vi "Metadata to FITS file header.vi"() -> ()   [LabVIEW 2023]
uses:
  gfitsio.lvlib
  gfitsio-write-key-double.vi
  gfitsio-write-key-string.vi
  cfitsio-bitpix.ctl
  gfitsio-read-image-subset-i16-2d.vi
  gfitsio-write-key-integer.vi
  gfitsio-write-image-subset-i16-2d.vi
  gfitsio-read-key-double.vi
  subvi/Git/GIT Data.ctl
  Data/MetaData/Typedef/MetaData.ctl
panel:
  out "concatenated string":string
  out "value":dbl
  out "header":string[](array[string])
  in  "MetaData":T1={"Test Name"="FPA CPT", "WOA Number"="0222", "User Name"="OCIfpa", "Operator"="Steve Marlow", "DUT SN"="SN0001", "Machine Name"="NI01", "OS Version"="WinNT 7", "Location"="HFF", "Top VI LV Rev."=123, "Lab Temperature"=23.5, "Lab Humidity"=49.9, "GIT"=[]}
  in  "file path":path=path "C:/Users/smarlow/Documents/FPA/gain_00014ms_1600x200_0017.fits"
  out "error out":errorcluster
  out "data":i16[][](array[numeric])
  out "Image":T3(plugin-control)
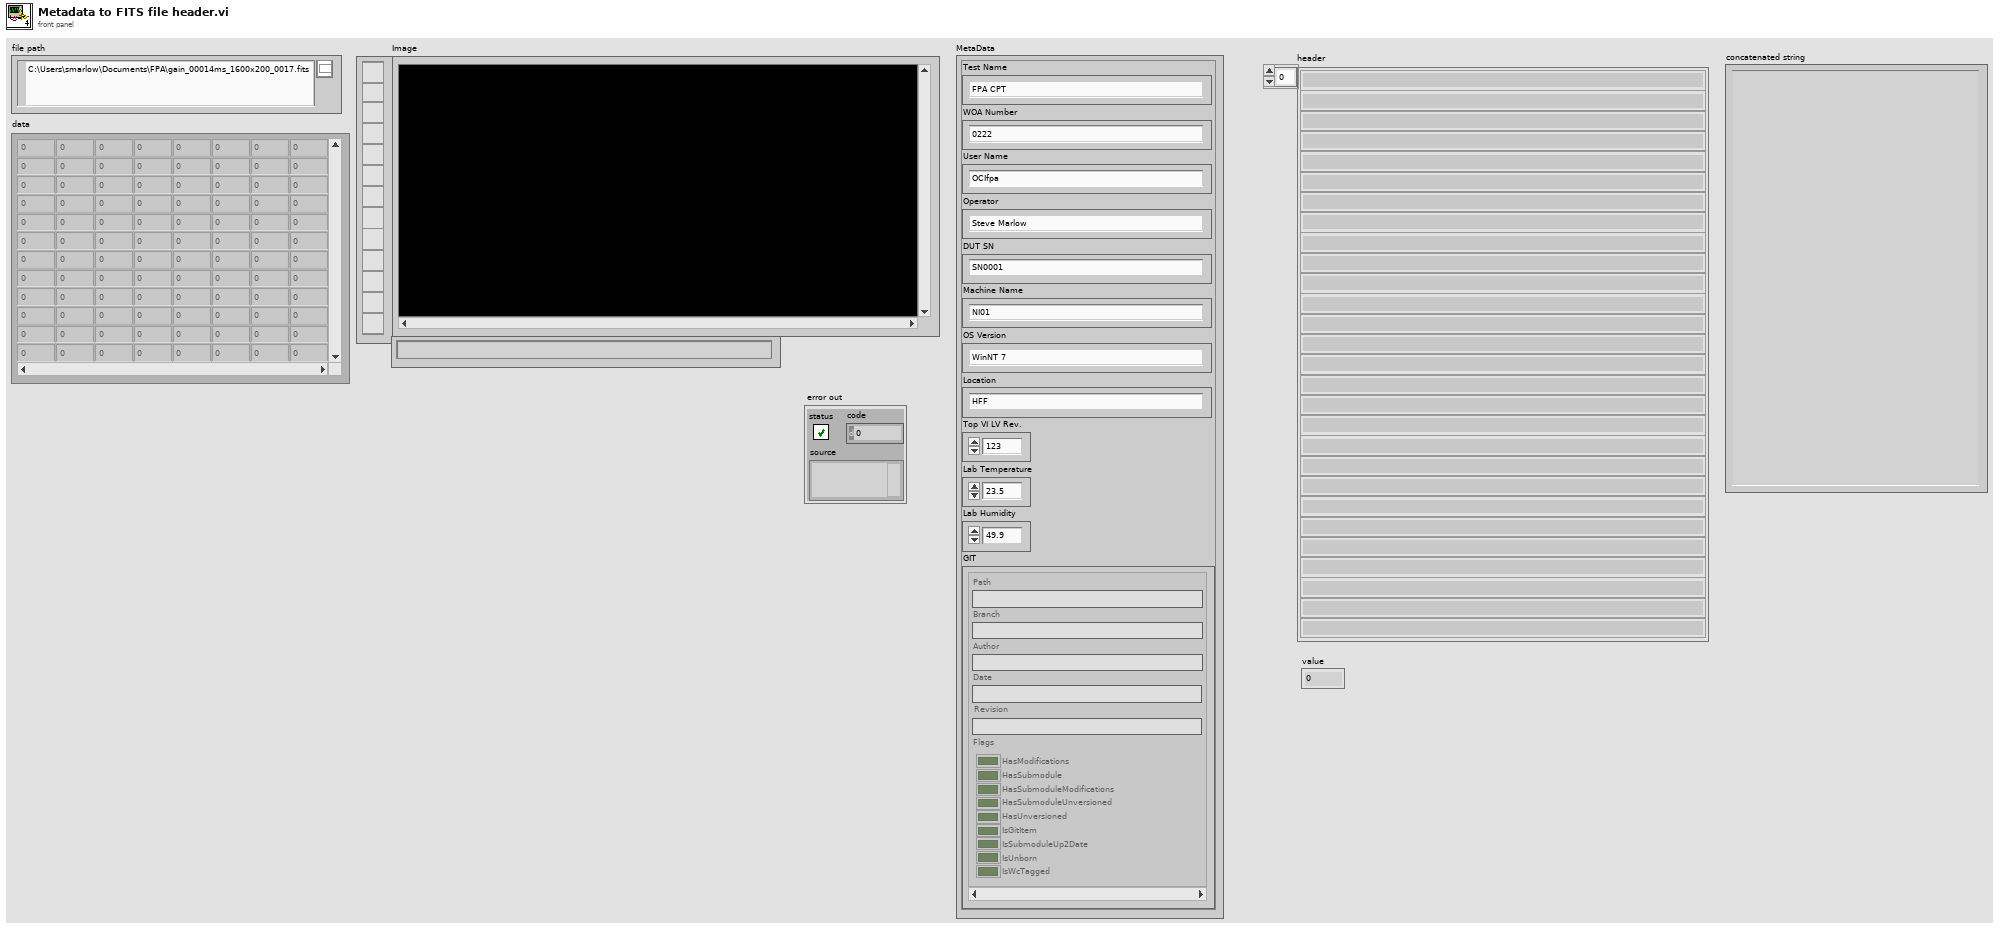
[diagram p1: front panel]
types:
  T1 = typedef "Data.MetaData.lvclass/MetaData.ctl" = cluster{"Test Name":string, "WOA Number":string, "User Name":string, "Operator":string, "DUT SN":string, "Machine Name":string, "OS Version":string, "Location":string, "Top VI LV Rev.":u32, "Lab Temperature":dbl, "Lab Humidity":dbl, "GIT":T2[]}
  T2 = typedef "GIT Data.ctl" = cluster{"Path":string, "Branch":string, "Author":string, "Date":string, "Revision":string, "Flags":cluster{"HasModifications":bool, "HasSubmodule":bool, "HasSubmoduleModifications":bool, "HasSubmoduleUnversioned":bool, "HasUnversioned":bool, "IsGitItem":bool, "IsSubmoduleUp2Date":bool, "IsUnborn":bool, "IsWcTagged":bool}}
  T3 = typedef "IMAQ Image.ctl" = refnum<image>
  T4 = typedef "gfitsio.lvlib/cfitsio-bitpix.ctl" = i32
  T5 = enum16{"open", "open or create", "create or replace", "create", "open (read only)"}
  T6 = typedef "Image Type" = u32
  T7 = typedef "gfitsio.lvlib/gfitsio-refnum.ctl" = refnum<k1>
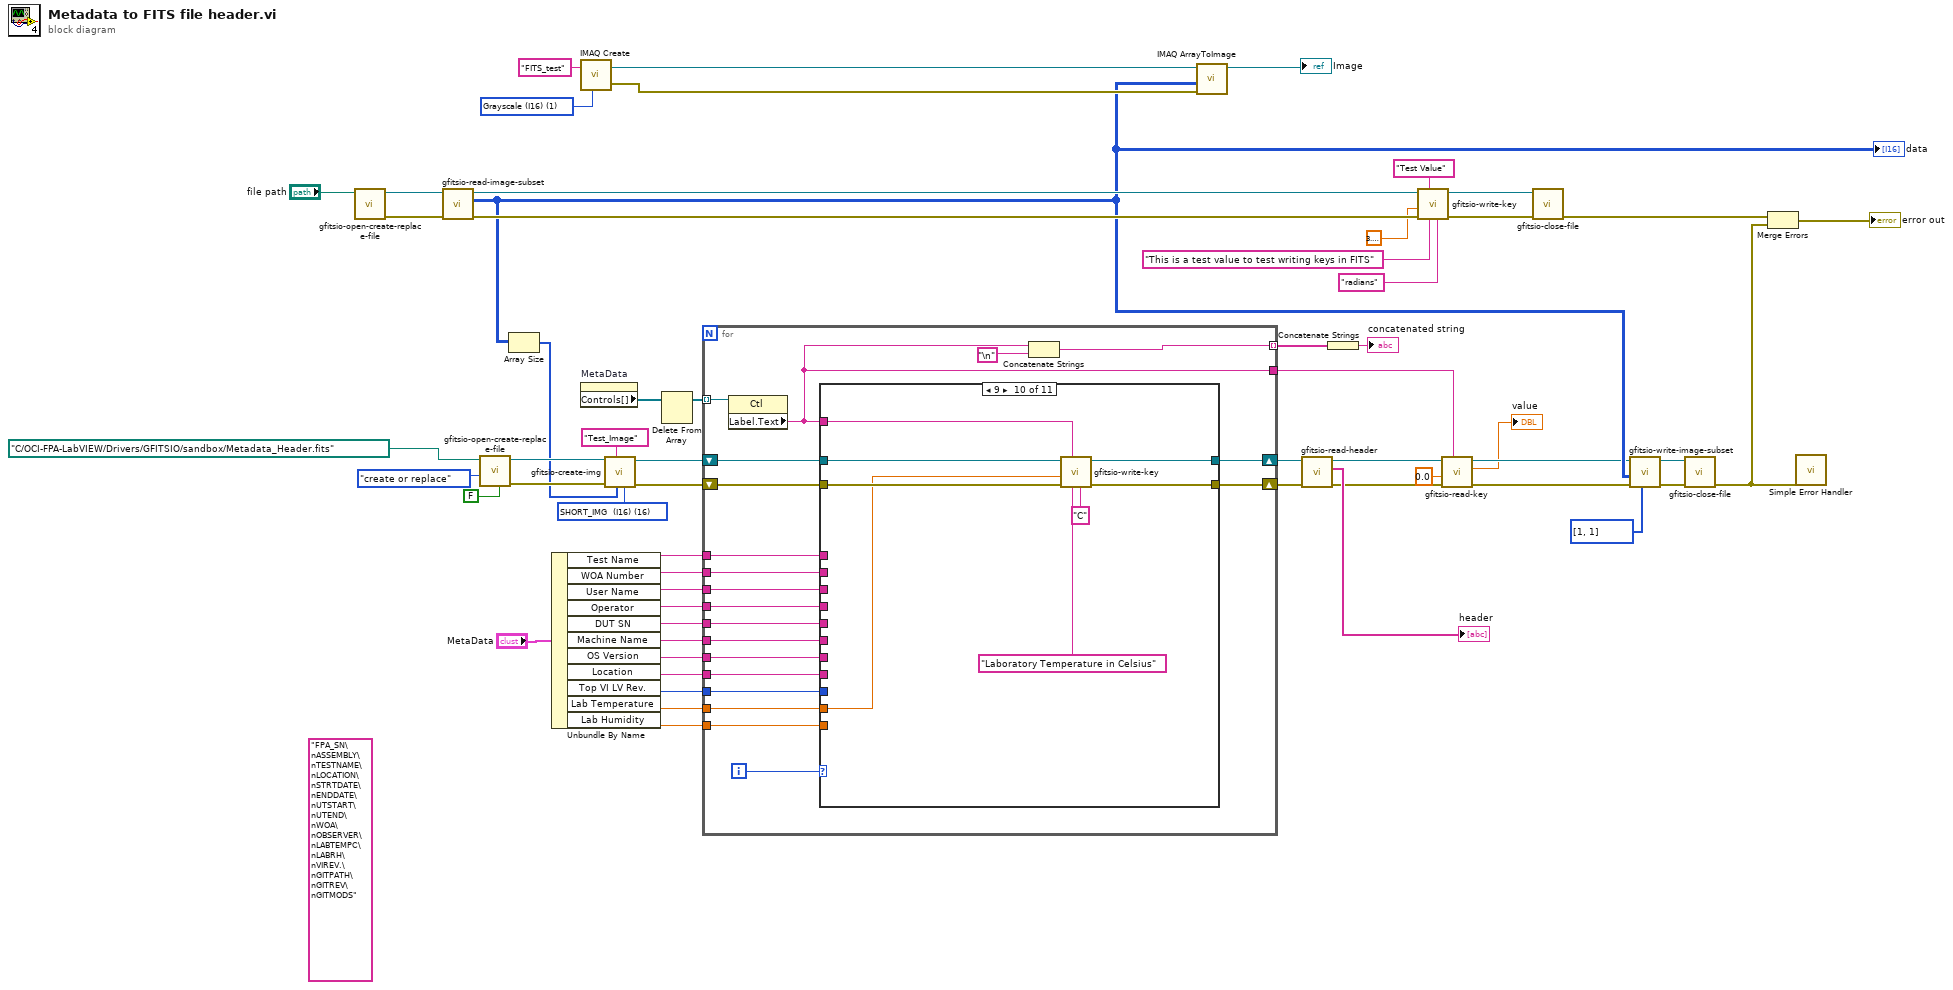
[diagram p0: block diagram]
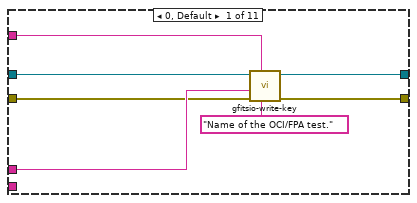
[diagram p2: hidden frame]
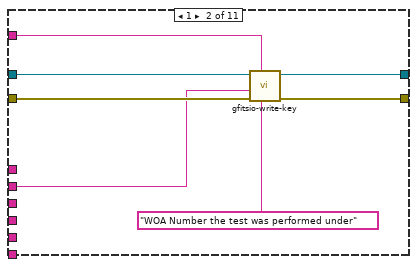
[diagram p3: hidden frame]
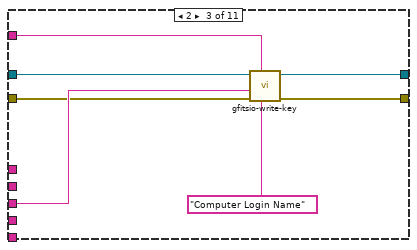
[diagram p4: hidden frame]
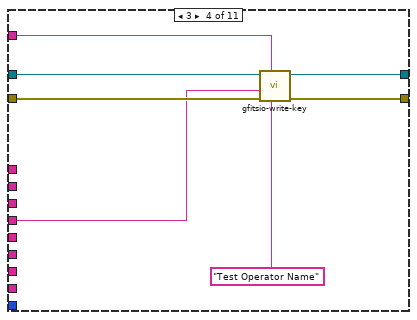
[diagram p5: hidden frame]
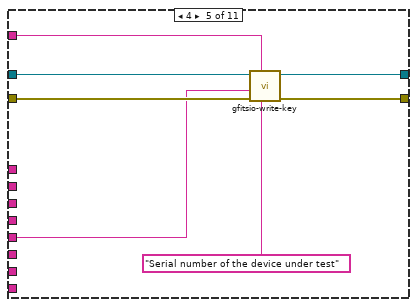
[diagram p6: hidden frame]
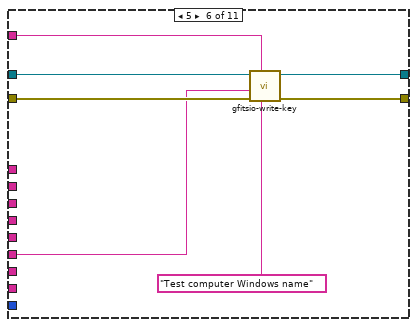
[diagram p7: hidden frame]
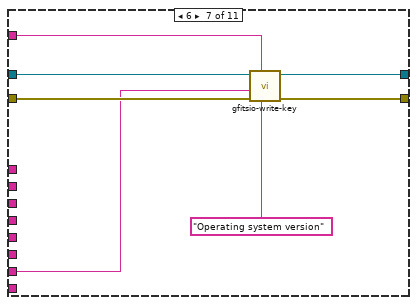
[diagram p8: hidden frame]
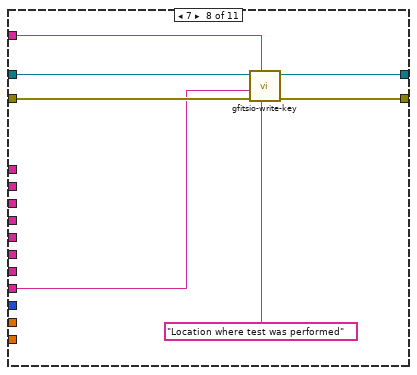
[diagram p9: hidden frame]
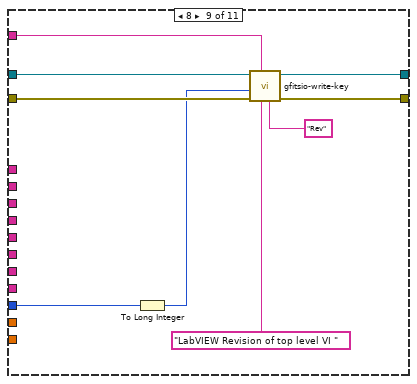
[diagram p10: hidden frame]
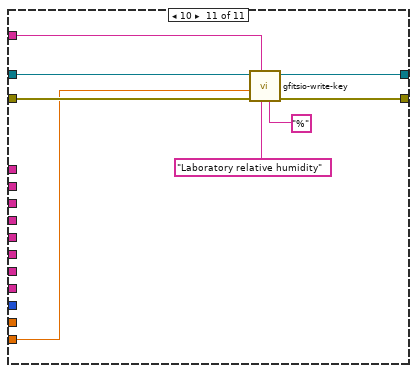
[diagram p11: hidden frame]
diagram:
  (unwired) "FPA_SN\nASSEMBLY\nTESTNAME\nLOCATION\nSTRTDATE\nENDDATE\nUTSTART\nUTEND\nWOA\nOBSERVER\nLABTEMPC\nLABRH\nVIREV.\nGITPATH\nGITREV\nGITMODS" ("format string")
  w19 = T4 16 items=["<invalid type>"=0, "BYTE_IMG  (U8)"=8, "SHORT_IMG  (I16)"=16, "USHORT_IMG  (U16)"=20, "LONG_IMG  (I32)"=32, "ULONG_IMG  (U32)"=40, "FLOAT_IMG  (SGL)"=-32, "DOUBLE_IMG  (DBL)"=-64] ("image data type")
  w54 = T6 1 items=["Grayscale (U8)", "Grayscale (I16)", "Grayscale (SGL)", "Complex (CSG)", "RGB (U32)", "HSL (U32)", "RGB (U64)", "Grayscale (U16)"] ("Image Type")
  n1 = call "gfitsio-open-create-replace-file.vi"("file path (dialog if empty)"="file path") -> ("error out"=w58:errorcluster, "gfits refnum"=w59:T7)  [unwired: 8 in, 1 out]
  n2 = call-poly "gfitsio-read-image-subset.vi"("error in (no error)"=w58, "gfits refnum"=w59) -> ("error out"=w48:errorcluster, "data"=w11:i16[][], "dup gfits refnum"=w56:T7)  [unwired: 7 in]
  "data" <- w11
  n3 = call "gfitsio-open-create-replace-file.vi"("advisory dialog? (display:T)"=FALSE, "function (open)"=T5."create or replace", "file path (dialog if empty)"=path "C:/OCI-FPA-LabVIEW/Drivers/GFITSIO/sandbox/Metadata_Header.fits") -> ("error out"=w13:errorcluster, "gfits refnum"=w15:T7)  [unwired: 6 in, 1 out]
  n4 = Array Size(array=w11) -> (size(s)=w10:i32[])
  n5 = Unbundle By Name("MetaData") -> ("Test Name"=w37:string, "WOA Number"=w36:string, "User Name"=w35:string, "Operator"=w34:string, "DUT SN"=w33:string, "Machine Name"=w32:string, "OS Version"=w31:string, "Location"=w30:string, "Top VI LV Rev."=w29:u32, "Lab Temperature"=w28:dbl, "Lab Humidity"=w27:dbl)
  n6 = call "IMAQ Create"("Image Name"="FITS_test", "Image Type"=w54) -> ("New Image"=w52:T3, "error out"=w51:errorcluster)  [unwired: 3 in]
  n7 = property on="MetaData" class="Clust (strict)"() -> ("Controls[]"=w39:refnum<vi>[])  [unwired: 2 in, 2 out]
  n8 = call "gfitsio-create-img.vi"("image data type"=w19, "naxes"=w10, "extname"="Test_Image", "error in (no error)"=w13, "gfits refnum"=w15) -> ("error out"=w12:errorcluster, "dup gfits refnum"=w14:T7)  [unwired: 5 in]
  n9 = Delete From Array(array=w39) -> (array with subset deleted=w38:refnum<vi>[])  [unwired: 2 in, 1 out]
  n10 = for {
    tunnel: w38 -> [w79] mode=indexing
    shift-right: [w76] -> w23
    shift-left: w14 -> [w77]
    tunnel: w37 -> [w75]
    tunnel: w36 -> [w74]
    tunnel: w35 -> [w73]
    shift-right: [w71] -> w22
    shift-left: w12 -> [w72]
    tunnel: w34 -> [w70]
    tunnel: w33 -> [w69]
    tunnel: w32 -> [w68]
    tunnel: w31 -> [w67]
    tunnel: w30 -> [w66]
    tunnel: w29 -> [w65]
    tunnel: w28 -> [w64]
    tunnel: w27 -> [w63]
    tunnel: [w62] -> w7
    tunnel: [w61] -> w2 mode=indexing
    i -> [w78]
    n11 = property class="Ctl"(reference=w79) -> ("Label.Text"=w62:string)  [unwired: 1 in, 2 out]
    n12 = case shown="9" w78 {
      tunnel: w77 -> [w86 w93 w100 w107 w114 w121 w128 w135 w144 w152 w160]
      tunnel: [w85 w92 w99 w106 w113 w120 w127 w134 w143 w151 w159] -> w76
      tunnel: w62 -> [w84 w91 w98 w105 w112 w119 w126 w133 w142 w150 w158]
      tunnel: w75 -> [w83 _ _ _ _ _ _ _ _ _ _]
      tunnel: w74 -> [_ w88 _ _ _ _ _ _ _ _ _]
      tunnel: w73 -> [_ _ w97 _ _ _ _ _ _ _ _]
      tunnel: w72 -> [w82 w90 w96 w104 w111 w118 w125 w132 w141 w149 w157]
      tunnel: [w81 w89 w95 w103 w110 w117 w124 w131 w140 w148 w156] -> w71
      tunnel: w70 -> [_ _ _ w102 _ _ _ _ _ _ _]
      tunnel: w69 -> [_ _ _ _ w109 _ _ _ _ _ _]
      tunnel: w68 -> [_ _ _ _ _ w116 _ _ _ _ _]
      tunnel: w67 -> [_ _ _ _ _ _ w123 _ _ _ _]
      tunnel: w66 -> [_ _ _ _ _ _ _ w130 _ _ _]
      tunnel: w65 -> [_ _ _ _ _ _ _ _ w139 _ _]
      tunnel: w64 -> [_ _ _ _ _ _ _ _ _ w146 _]
      tunnel: w63 -> [_ _ _ _ _ _ _ _ _ _ w155]
      frame 0, Default {
        n13 = call-poly "gfitsio-write-key.vi"("comment"="Name of the OCI/FPA test.", "keyname"=w84, "error in (no error)"=w82, "value"=w83, "gfits refnum"=w86) -> ("error out"=w81:errorcluster, "dup gfits refnum"=w85:T7)  [unwired: 5 in]
      }
      frame 1 {
        n14 = call-poly "gfitsio-write-key.vi"("comment"="WOA Number the test was performed under", "keyname"=w91, "error in (no error)"=w90, "value"=w88, "gfits refnum"=w93) -> ("error out"=w89:errorcluster, "dup gfits refnum"=w92:T7)  [unwired: 5 in]
      }
      frame 2 {
        n15 = call-poly "gfitsio-write-key.vi"("comment"="Computer Login Name", "keyname"=w98, "error in (no error)"=w96, "value"=w97, "gfits refnum"=w100) -> ("error out"=w95:errorcluster, "dup gfits refnum"=w99:T7)  [unwired: 5 in]
      }
      frame 3 {
        n16 = call-poly "gfitsio-write-key.vi"("comment"="Test Operator Name", "keyname"=w105, "error in (no error)"=w104, "value"=w102, "gfits refnum"=w107) -> ("error out"=w103:errorcluster, "dup gfits refnum"=w106:T7)  [unwired: 5 in]
      }
      frame 4 {
        n17 = call-poly "gfitsio-write-key.vi"("comment"="Serial number of the device under test", "keyname"=w112, "error in (no error)"=w111, "value"=w109, "gfits refnum"=w114) -> ("error out"=w110:errorcluster, "dup gfits refnum"=w113:T7)  [unwired: 5 in]
      }
      frame 5 {
        n18 = call-poly "gfitsio-write-key.vi"("comment"="Test computer Windows name", "keyname"=w119, "error in (no error)"=w118, "value"=w116, "gfits refnum"=w121) -> ("error out"=w117:errorcluster, "dup gfits refnum"=w120:T7)  [unwired: 5 in]
      }
      frame 6 {
        n19 = call-poly "gfitsio-write-key.vi"("comment"="Operating system version", "keyname"=w126, "error in (no error)"=w125, "value"=w123, "gfits refnum"=w128) -> ("error out"=w124:errorcluster, "dup gfits refnum"=w127:T7)  [unwired: 5 in]
      }
      frame 7 {
        n20 = call-poly "gfitsio-write-key.vi"("comment"="Location where test was performed", "keyname"=w133, "error in (no error)"=w132, "value"=w130, "gfits refnum"=w135) -> ("error out"=w131:errorcluster, "dup gfits refnum"=w134:T7)  [unwired: 5 in]
      }
      frame 8 {
        n21 = To Long Integer(number=w139) -> (32bit integer=w138:i32)
        n22 = call-poly "gfitsio-write-key.vi"("units"="Rev", "comment"="LabVIEW Revision of top level VI ", "keyname"=w142, "error in (no error)"=w141, "value"=w138, "gfits refnum"=w144) -> ("error out"=w140:errorcluster, "dup gfits refnum"=w143:T7)  [unwired: 4 in]
      }
      frame 9 {
        n23 = call-poly "gfitsio-write-key.vi"("units"="C", "comment"="Laboratory Temperature in Celsius", "keyname"=w150, "error in (no error)"=w149, "value"=w146, "gfits refnum"=w152) -> ("error out"=w148:errorcluster, "dup gfits refnum"=w151:T7)  [unwired: 4 in]
      }
      frame 10 {
        n24 = call-poly "gfitsio-write-key.vi"("units"="%", "comment"="Laboratory relative humidity", "keyname"=w158, "error in (no error)"=w157, "value"=w155, "gfits refnum"=w160) -> ("error out"=w156:errorcluster, "dup gfits refnum"=w159:T7)  [unwired: 4 in]
      }
    }
    n25 = Concatenate Strings(w62, "\n") -> (w61:string)
  }
  n26 = call "IMAQ ArrayToImage"("error in (no error)"=w51, "Image Pixels (I16)"=w11, "Image"=w52) -> ("Image Out"=→"Image":T3)  [unwired: 7 in, 1 out]
  n27 = call "gfitsio-read-header.vi"("error in (no error)"=w22, "gfits refnum"=w23) -> ("error out"=w8:errorcluster, "header"=→"header":string[], "dup gfits refnum"=w9:T7)  [unwired: 7 in]
  n28 = Concatenate Strings(w2) -> (→"concatenated string":string)
  n29 = call-poly "gfitsio-write-key.vi"("units"="radians", "comment"="This is a test value to test writing keys in FITS", "keyname"="Test Value", "error in (no error)"=w48, "value"=3.141592653589793, "gfits refnum"=w56) -> ("error out"=w47:errorcluster, "dup gfits refnum"=w49:T7)  [unwired: 4 in]
  n30 = call-poly "gfitsio-read-key.vi"("keyname"=w7, "error in (no error)"=w8, "default value"=0.0, "gfits refnum"=w9) -> ("error out"=w5:errorcluster, "value"=→"value":dbl, "dup gfits refnum"=w6:T7)  [unwired: 3 in, 2 out]
  n31 = call "gfitsio-close-file.vi"("error in (no error)"=w47, "gfits refnum"=w49) -> ("error out"=w55:errorcluster)  [unwired: 8 in, 1 out]
  n32 = call-poly "gfitsio-write-image-subset.vi"("fpixel"=i32[] [1, 1], "error in (no error)"=w5, "data"=w11, "gfits refnum"=w6) -> ("error out"=w17:errorcluster, "dup gfits refnum"=w16:T7)  [unwired: 6 in]
  n33 = call "gfitsio-close-file.vi"("error in (no error)"=w17, "gfits refnum"=w16) -> ("error out"=w24:errorcluster)  [unwired: 8 in, 1 out]
  n34 = Merge Errors(w55, w24) -> (→"error out":errorcluster)
  n35 = call <vilib>:"Simple Error Handler.vi"("error in (no error)"=w24) -> ()  [unwired: 4 in, 5 out]
